vi "根据ini文件刷新下拉框.vi"(0 "refnum":T1, 1 "Ring引用句柄":refnum<vi>, 3 "error in (no error)":errorcluster caption="错误输入（无错误）") -> (7 "引用句柄输出":T1 caption="refnum out", 10 "错误输出":errorcluster)   [LabVIEW 2015]
uses:
  <vilib>/Utility/config.llb/Config Data RefNum.ctl
  <vilib>/Utility/config.llb/NI_LVConfig.lvlib
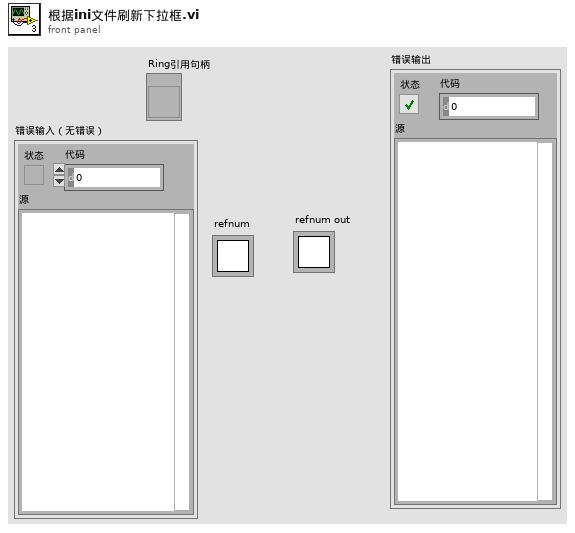
[diagram p1: front panel]
types:
  T1 = typedef "NI_LVConfig.lvlib/Config Data RefNum.ctl" = refnum<k1>
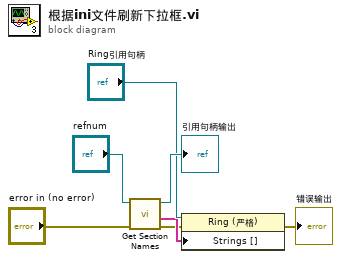
[diagram p0: block diagram]
diagram:
  n1 = call <vilib>:"Get Section Names.vi"("error in (no error)"="error in (no error)", "refnum"="refnum") -> ("error out"=w3:errorcluster, "section names"=w4:string[], "refnum out"=→"引用句柄输出":T1)  [unwired: 7 in]
  n2 = property class="Ring (严格)"(reference="Ring引用句柄", error in=w3, "Strings []"=w4) -> (error out=→"错误输出":errorcluster)  [unwired: 1 out]
